vi "rad_Open System Config Session.vi"(7 "Access requirement (admin unless unlocked)":T3=enum."Admin unless unlocked", 8 "error in (no error)":errorcluster, 11 "Target settings":T1={"Hostname"="", "Serial number"="", "Product name"="", "Product code"=0, "System status"="", "Credential type"=enum."None/Unlocked", "User added?"=FALSE, "Primary NIC"={"MAC address"="", "IP Address Request Mode"=2, "IP address"="", "Subnet mask"="", "Gateway"="", "DNS server"=""}} {"Primary NIC"."IP Address Request Mode" items=["Static"=1, "DHCP/Link-Local"=2, "Link-Local Only"=4, "DHCP Only"=8]}) -> (0 "error out":errorcluster, 1 "Password out":string, 2 "Cancelled":bool, 3 "Session out":refnum<k21>)   [LabVIEW 2014]
uses:
  Targets/TypeDefs/rad_Initialize Access Types.ctl
  Targets/TypeDefs/rad_Target Information.ctl
  Targets/TypeDefs/rad_Target Network Settings.ctl
  rad_Globals.vi
  <vilib>/nisyscfg/Close (System).vi
  <vilib>/nisyscfg/nisyscfg.lvlib
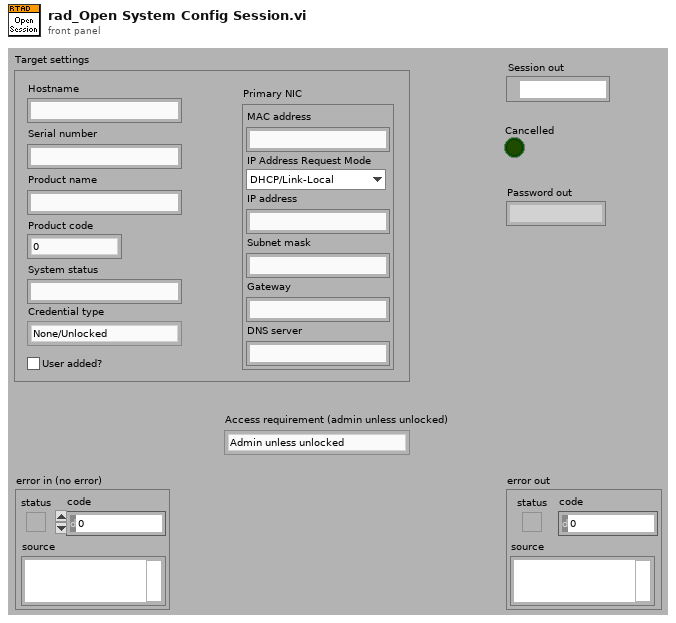
[diagram p1: front panel]
types:
  T1 = typedef "rad_Target Information.ctl" = cluster{"Hostname":string, "Serial number":string, "Product name":string, "Product code":i32, "System status":string, "Credential type":enum16{"None/Unlocked", "FTP Password", "NIAuth Credentials"}, "User added?":bool, "Primary NIC":T2}
  T2 = typedef "rad_Target Network Settings.ctl" = cluster{"MAC address":string, "IP Address Request Mode":i32, "IP address":string, "Subnet mask":string, "Gateway":string, "DNS server":string}
  T3 = typedef "rad_Initialize Access Types.ctl" = enum16{"Anonymous read-only", "Admin unless unlocked", "Admin always"}
  T4 = enum16{"None/Unlocked", "FTP Password", "NIAuth Credentials"}
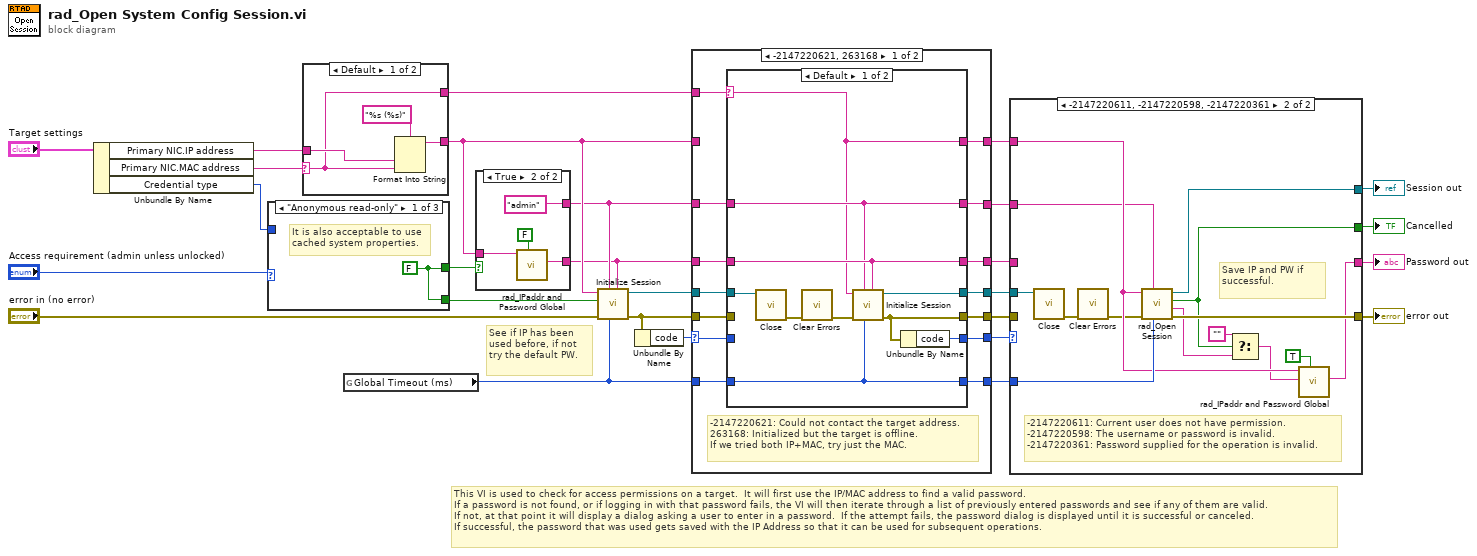
[diagram p0: block diagram]
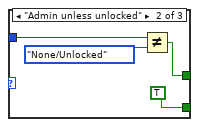
[diagram p4: hidden frame]
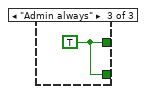
[diagram p5: hidden frame]
diagram:
  # "This VI is used to check for access permissions on a target.  It will first use the IP/MAC address to find a valid password. \nIf a password is not found, or if logging in with that password fails, the VI will then iterate through a list of previously entered passwords and see if any of them are valid.\nIf not, at that point it will display a dialog asking a user to enter in a password.  If the attempt fails, the password dialog is displayed until it is successful or canceled. \nIf successful, the password that was used gets saved with the IP Address so that it can be used for subsequent operations."
  # "See if IP has been used before, if not try the default PW."
  n1 = Unbundle By Name("Target settings") -> ("Primary NIC.IP address"=w20:string, "Primary NIC.MAC address"=w21:string, "Credential type"=w18:T4)
  n2 = case shown="\"Anonymous read-only\"" "Access requirement (admin unless unlocked)" {
    tunnel: w18 -> [_ w31 _]
    tunnel: [w28 w30 w33] -> w17
    tunnel: [w28 TRUE w33] -> w16
    frame "Anonymous read-only" {
      w28 = FALSE
      # "It is also acceptable to use\ncached system properties."
    }
    frame "Admin unless unlocked" {
      n3 = Not Equal?(x=w31, y=T4."None/Unlocked") -> (x != y?=w30:bool)
    }
    frame "Admin always" {
      w33 = TRUE
    }
  }
  n4 = case shown="Default" w21 {
    selector: w21 -> [w34 _]
    tunnel: w20 -> [w35 w38]
    tunnel: [w36 w38] -> w13
    tunnel: [w34 _] -> w2
    frame Default {
      n5 = Format Into String(format string="%s (%s)", w35, w34) -> (resulting string=w36:string)  [unwired: 2 in, 1 out]
    }
    frame "" {
    }
  }
  n6 = global read "rad_Globals.vi" "Global Timeout (ms)"() -> (w1:u32)
  n7 = case shown="True" w17 {
    tunnel: [_ w41] -> w9
    tunnel: w13 -> [_ w40]
    tunnel: [_ "admin"] -> w11
    frame False {
    }
    frame True {
      n8 = call "rad_IPaddr and Password Global.vi"("Read(F)/Write(T)"=FALSE, "IP/MAC Address"=w40) -> ("Password"=w41:string)  [unwired: 8 in, 1 out]
    }
  }
  n9 = call <vilib>:"Initialize Session.vi"("Password"=w9, "Connect Timeout (4000 ms)"=w1, "User Name"=w11, "error in (no error)"="error in (no error)", "Force Property Refresh (T)"=w16, "Target (localhost)"=w13) -> ("error out"=w5:errorcluster, "Session out"=w7:refnum<k21>)  [unwired: 4 in]
  n10 = Unbundle By Name(w5) -> ("code"=w15:i32)
  n11 = case shown="-2147220621, 263168" w15 {
    selector: w15 -> [w43 w77]
    tunnel: [w51 w77] -> w14
    tunnel: w13 -> [_ w76]
    tunnel: [w45 w76] -> w12
    tunnel: w11 -> [w50 w75]
    tunnel: [w46 w75] -> w10
    tunnel: w9 -> [w49 w74]
    tunnel: [w47 w74] -> w8
    tunnel: w7 -> [w55 w73]
    tunnel: [w54 w73] -> w6
    tunnel: w5 -> [w53 w72]
    tunnel: [w52 w72] -> w4
    tunnel: w1 -> [w48 w71]
    tunnel: [w44 w71] -> w3
    tunnel: w2 -> [w56 _]
    frame -2147220621, 263168 {
      # "-2147220621: Could not contact the target address.\n263168: Initialized but the target is offline.\nIf we tried both IP+MAC, try just the MAC."
      n12 = case shown="Default" w56 {
        selector: w56 -> [w58 _]
        tunnel: w55 -> [w66 w70]
        tunnel: [w61 w70] -> w54
        tunnel: w53 -> [_ w69]
        tunnel: [w63 w69] -> w52
        tunnel: [w62 w68] -> w51
        tunnel: w50 -> [w59 _]
        tunnel: w49 -> [w60 w67]
        tunnel: w48 -> [w57 _]
        tunnel: [w60 w67] -> w47
        tunnel: [w59 _] -> w46
        tunnel: [w58 _] -> w45
        tunnel: [w57 _] -> w44
        tunnel: w43 -> [_ w68]
        frame Default {
          n13 = call-poly <vilib>:"Close.vi"("Session in"=w66) -> ("error out"=w65:errorcluster)  [unwired: 10 in]
          n14 = call <vilib>:"Clear Errors.vi"("error in (no error)"=w65) -> ("error out"=w64:errorcluster)  [unwired: 5 in, 1 out]
          n15 = call <vilib>:"Initialize Session.vi"("Password"=w60, "Connect Timeout (4000 ms)"=w57, "User Name"=w59, "error in (no error)"=w64, "Target (localhost)"=w58) -> ("error out"=w63:errorcluster, "Session out"=w61:refnum<k21>)  [unwired: 5 in]
          n16 = Unbundle By Name(w63) -> ("code"=w62:i32)
        }
        frame "" {
        }
      }
    }
    frame Default {
    }
  }
  n17 = case shown="-2147220611, -2147220598, -2147220361" w14 {
    tunnel: w4 -> [w80 _]
    tunnel: [w80 w92] -> w27
    tunnel: w6 -> [w79 w94]
    tunnel: [w79 w93] -> w24
    tunnel: w12 -> [_ w90]
    tunnel: [_ w84] -> w26
    tunnel: w3 -> [_ w91]
    tunnel: [w78 w89] -> w23
    tunnel: w8 -> [w78 _]
    tunnel: w10 -> [_ w86]
    frame Default {
    }
    frame -2147220611, -2147220598, -2147220361 {
      # "Save IP and PW if successful."
      # "-2147220611: Current user does not have permission.\n-2147220598: The username or password is invalid.\n-2147220361: Password supplied for the operation is invalid."
      n18 = call-poly <vilib>:"Close.vi"("Session in"=w94) -> ("error out"=w88:errorcluster)  [unwired: 10 in]
      n19 = call <vilib>:"Clear Errors.vi"("error in (no error)"=w88) -> ("error out"=w87:errorcluster)  [unwired: 5 in, 1 out]
      n20 = call "rad_Open Session.vi"("Timeout ms (4s)"=w91, "User name"=w86, "error in (no error)"=w87, "Target Address"=w90) -> ("error out"=w92:errorcluster, "Password Out"=w83:string, "Cancelled"=w84:bool, "session out"=w93:refnum<k21>)  [unwired: 4 in]
      n21 = Select(t="", s=w84, f=w83) -> (s? t:f=w82:string)
      n22 = call "rad_IPaddr and Password Global.vi"("Read(F)/Write(T)"=TRUE, "Password"=w82, "IP/MAC Address"=w90) -> ("Password"=w89:string)  [unwired: 7 in, 1 out]
    }
  }
  "error out" <- w27
  "Session out" <- w24
  "Cancelled" <- w26
  "Password out" <- w23
